vi "Configure Alternation Trigger (Edge).vi"(0 "VISA resource name":refnum<visa-resource-name>, 5 "Source Channel (0:Source A)":u16(ring) items=["Source A", "Source B"], 7 "Trigger Slope (0: Positive)":u16(ring) items=["Positive", "Negative"], 11 "error in (no error)":errorcluster) -> (4 "VISA resource name out":refnum<visa-resource-name>, 15 "error out":errorcluster)   [LabVIEW 2010, in "Agilent DSO1000 Series.lvlib"]
doc: "Configures the edge trigger under alternation trigger mode. An edge trigger occurs when the trigger signal has the slope that you specify with the \"Trigger Slope\" control."
uses:
  <instrlib>/Agilent DSO1000 Series/Agilent DSO1000 Series.lvlib
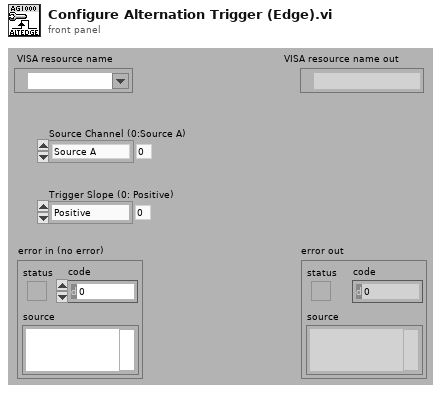
[diagram p1: front panel]
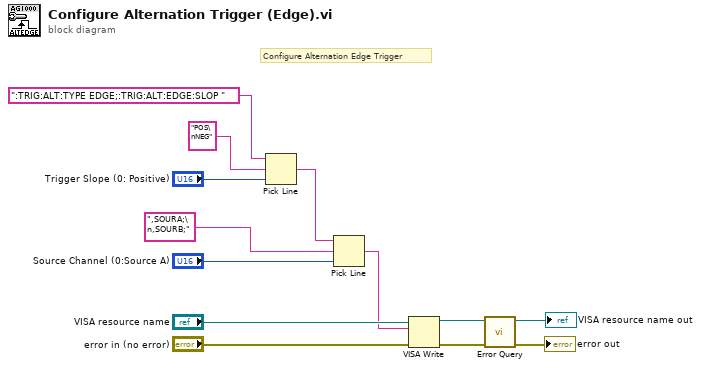
[diagram p0: block diagram]
diagram:
  # "Configure Alternation Edge Trigger"
  n1 = Pick Line(string ("")=":TRIG:ALT:TYPE EDGE;:TRIG:ALT:EDGE:SLOP ", multi-line string="POS\nNEG", line index="Trigger Slope (0: Positive)") -> (output string=w8:string)
  n2 = Pick Line(string ("")=w8, multi-line string=",SOURA;\n,SOURB;", line index="Source Channel (0:Source A)") -> (output string=w5:string)
  n3 = VISA Write(VISA resource name="VISA resource name", write buffer=w5, error in (no error)="error in (no error)") -> (VISA resource name out=w3:refnum<visa-resource-name>, error out=w4:errorcluster)  [unwired: 1 out]
  n4 = call <instrlib>:"Error Query.vi"("error in (no error)"=w4, "VISA resource name"=w3) -> ("error out"=→"error out":errorcluster, "VISA resource name out"=→"VISA resource name out":refnum<visa-resource-name>)  [unwired: 6 in, 2 out]
